vi "Close.vi"(8 "error in (no error)":errorcluster, 11 "CS++Message in":refnum<class "CS++Message.lvclass">) -> (0 "error out":errorcluster, 3 "CS++Message out":refnum<class "CS++Message.lvclass">)   [LabVIEW 2014, in "CS++Message.lvlib" / "CS++Message.lvclass"]
doc: "Removes the reference to the message."
uses:
  CS++Message.lvclass
  CS++Message.lvclass/CS++Message.ctl
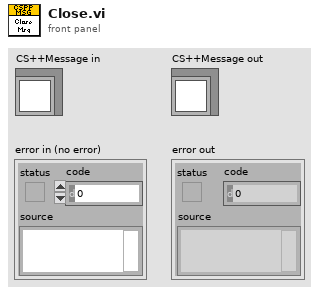
[diagram p1: front panel]
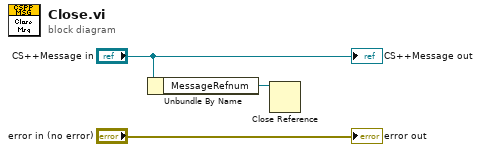
[diagram p0: block diagram]
diagram:
  n1 = Unbundle By Name("CS++Message in") -> ("MessageRefnum"=w1:refnum<vi>)
  n2 = Close Reference(reference=w1) -> ()  [unwired: 1 in, 1 out]
  "error out" <- "error in (no error)"
  "CS++Message out" <- "CS++Message in"
